vi "adam-4069-channel.vi"() -> ()   [LabVIEW 2021]
panel:
  in  "Stop Program":bool
  in  "Stop All":bool
  out "Status":string
  out "command":string
  in  "Channel Number":dbl=1.0 min=1.0 max=9.0 step=1.0
  in  "Channel Active":bool
  out "read buffer":string
  out "Bytes Written":u32
  out "Channel Active":bool
  out "error out":errorcluster
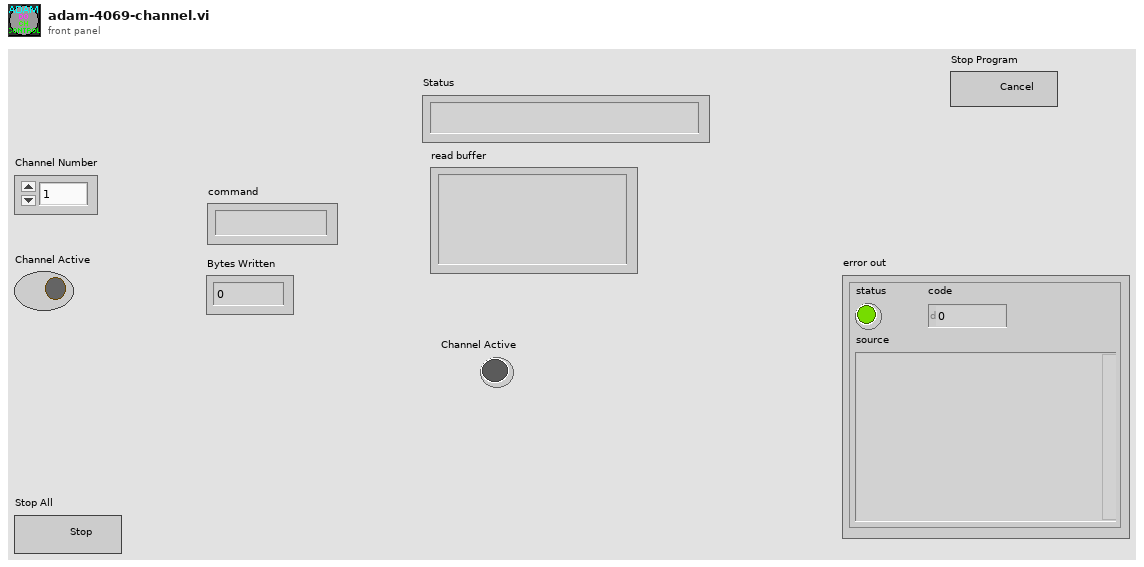
[diagram p1: front panel]
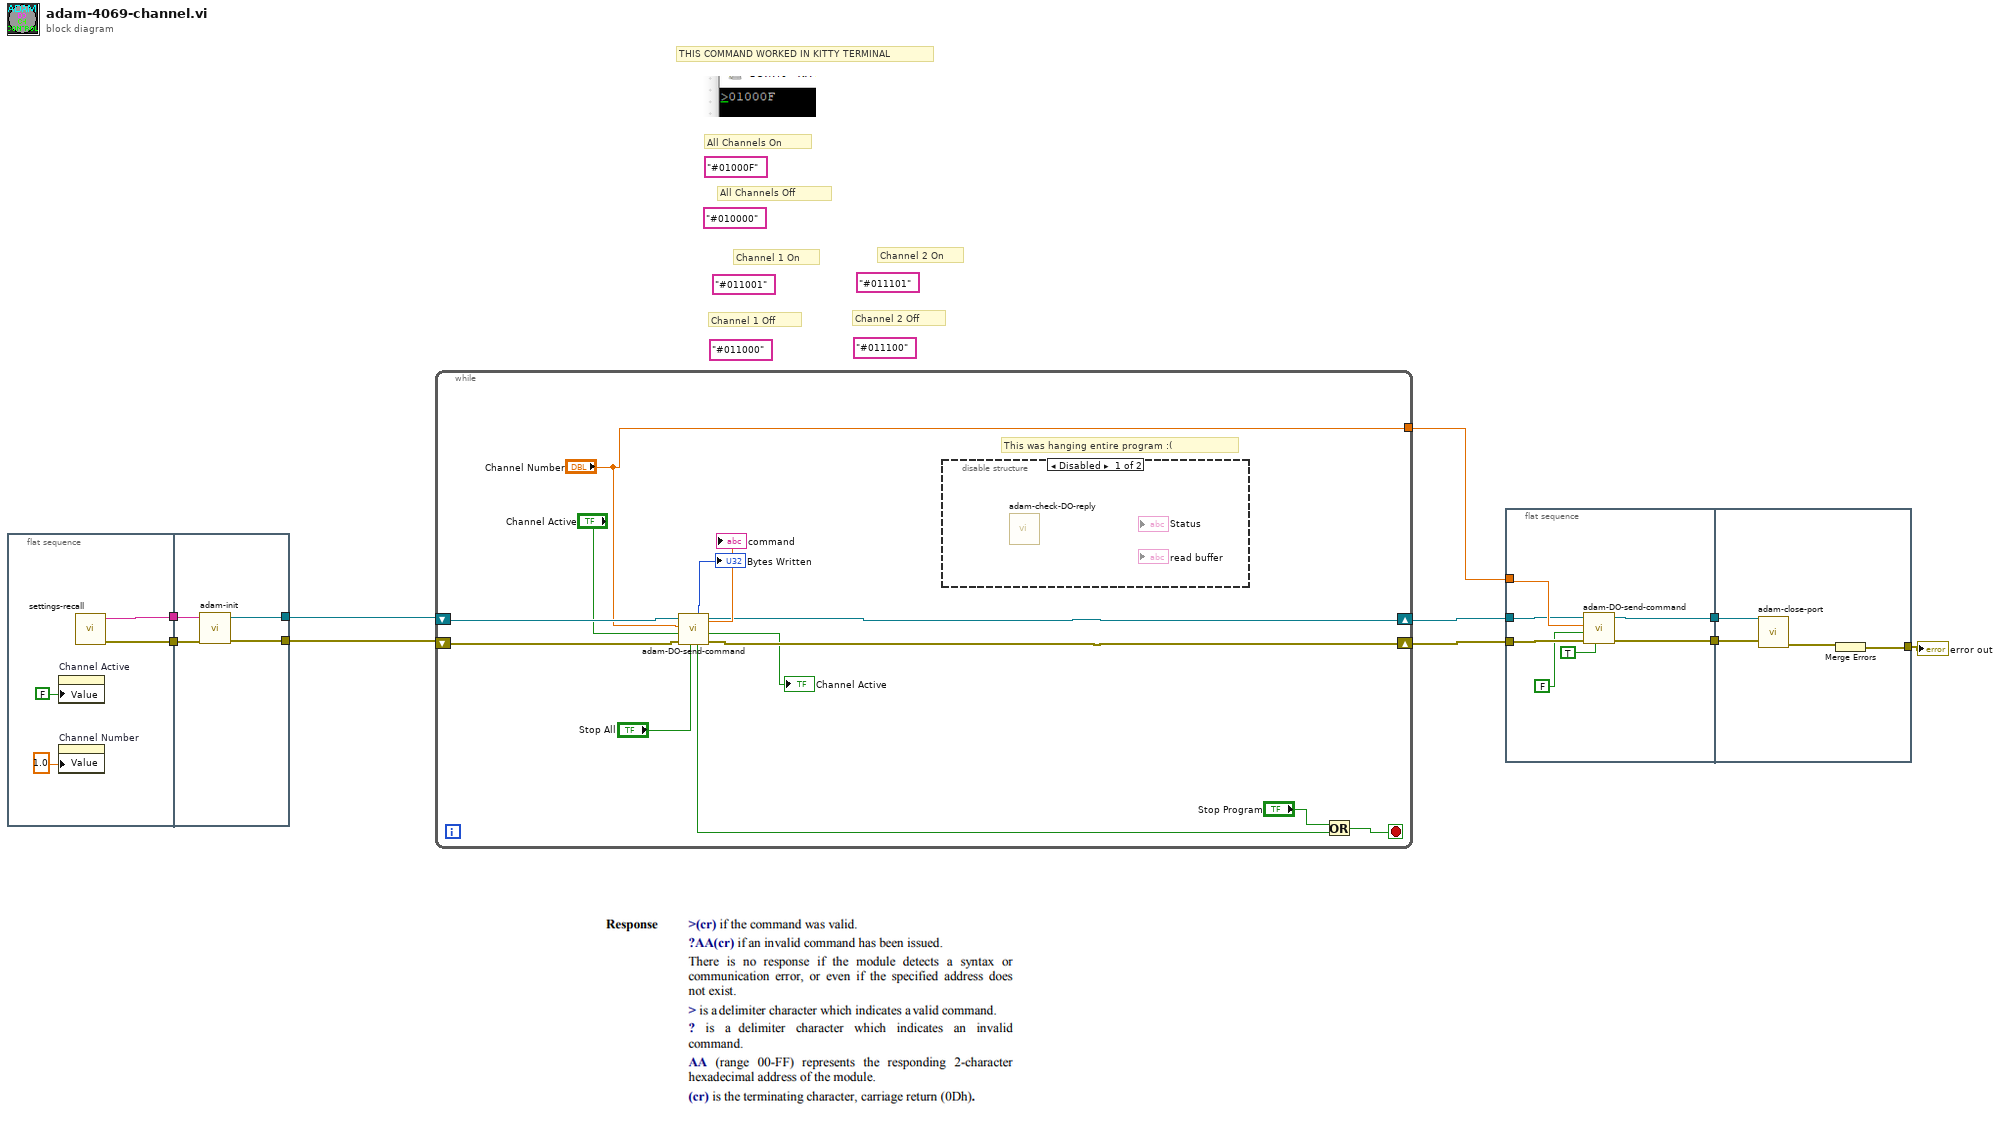
[diagram p0: block diagram]
diagram:
  (unwired) "#011101" ("write buffer")
  (unwired) "#011100" ("write buffer")
  (unwired) "#011001" ("write buffer")
  (unwired) "#011000" ("write buffer")
  (unwired) "#010000" ("write buffer")
  (unwired) "#01000F" ("write buffer")
  # "Channel 2 Off"
  # "Channel 2 On"
  # "Channel 1 Off"
  # "Channel 1 On"
  # "All Channels Off"
  # "All Channels On"
  # "THIS COMMAND WORKED IN KITTY TERMINAL"
  n1 = flat-sequence {
    tunnel: [w14] -> w7
    tunnel: [w13] -> w6
    tunnel: w7 -> [w17]
    tunnel: w6 -> [w18]
    tunnel: [w16] -> w5
    tunnel: [w15] -> w4
    frame #0 {
      n2 = property on="Channel Active" class="Bool (strict)"("Value"=FALSE ("Channel Active")) -> ()  [unwired: 2 in, 2 out]
      n3 = property on="Channel Number" class="DigNum (strict)"("Value"=1.0 ("Channel Number")) -> ()  [unwired: 2 in, 2 out]
      n4 = call "settings-recall.vi"() -> ("error out"=w13:errorcluster, "COM port"=w14:string)  [unwired: 9 in, 1 out]
    }
    frame #1 {
      n5 = call "adam-init.vi"("error in (no error)"=w18, "COM Port (COM10)"=w17) -> ("error out"=w15:errorcluster, "VISA resource name out"=w16:refnum<visa-resource-name>)  [unwired: 8 in]
    }
  }
  n6 = while {
    shift-right: [w21] -> w8
    shift-left: w5 -> [w31]
    shift-right: [w20] -> w10
    shift-left: w4 -> [w30]
    tunnel: ["Channel Number"] -> w9
    stop <- w24 stop-if-true
    # "This was hanging entire program :("
    n7 = call "adam-DO-send-command.vi"("Stop All"="Stop All", "error in (no error)"=w30, "Channel Active"="Channel Active", "Channel Number"="Channel Number", "VISA Refnum in"=w31) -> ("error out"=w20:errorcluster, "Desired State"=→"Channel Active":bool, "VISA Refnum out"=w21:refnum<visa-resource-name>, "STOPPED"=w25:bool, "Bytes Written"=→"Bytes Written":u32, "Device Address"=→"command":dbl)  [unwired: 1 out]
    n8 = disable-structure shown="Disabled" {
      frame Disabled {
        n9 = call "adam-check-DO-reply.vi"() -> ("Channel Active"=w32:bool)  [unwired: 7 in, 4 out]
      }
      frame Enabled {
      }
    }
    n10 = Or(x="Stop Program", y=w25) -> (x .or. y?=w24:bool)
  }
  n11 = flat-sequence {
    tunnel: w10 -> [w39]
    tunnel: w9 -> [w37]
    tunnel: w8 -> [w34]
    tunnel: [w38] -> w3
    tunnel: [w35] -> w2
    tunnel: w3 -> [w41]
    tunnel: w2 -> [w42]
    tunnel: [w40] -> w1
    frame #0 {
      n12 = call "adam-DO-send-command.vi"("Stop All"=TRUE, "error in (no error)"=w39, "Channel Active"=FALSE, "Channel Number"=w37, "VISA Refnum in"=w34) -> ("error out"=w35:errorcluster, "VISA Refnum out"=w38:refnum<visa-resource-name>)  [unwired: 1 in, 4 out]
    }
    frame #1 {
      n13 = call "adam-close-port.vi"("error in (no error)"=w42, "VISA Refnum in"=w41) -> ("error out"=w43:errorcluster)  [unwired: 9 in]
      n14 = Merge Errors(w43) -> (w40:errorcluster)
    }
  }
  "error out" <- w1
